vi "Drag and Drop - Initiating a Custom Drag.vi"() -> ()   [LabVIEW 2023]
doc: "Illustrates how to perform Drag and Drop operations from a custom source to a custom target."
panel:
  in  "Stop":bool
  in  "Plot to Drag":i32 min=0 max=4 step=1
  out "Target Waveform":dbl[](graph)
  out "Source Waveforms":dbl[][](graph)
  # "Overview: Demonstrates how to store the Mouse Down state and initiate custom drag operations when performing Drag and Drop actions with the Event Structure.\nInstructions:\n1. Run the VI.\n2. Specify a value for the Plot to Drag.\n3. Drag the plot area of the Source Waveforms graph to the Target Waveform graph. The specified Plot to Drag will appear in the Target Waveform.\n4. Click Stop to stop the VI."
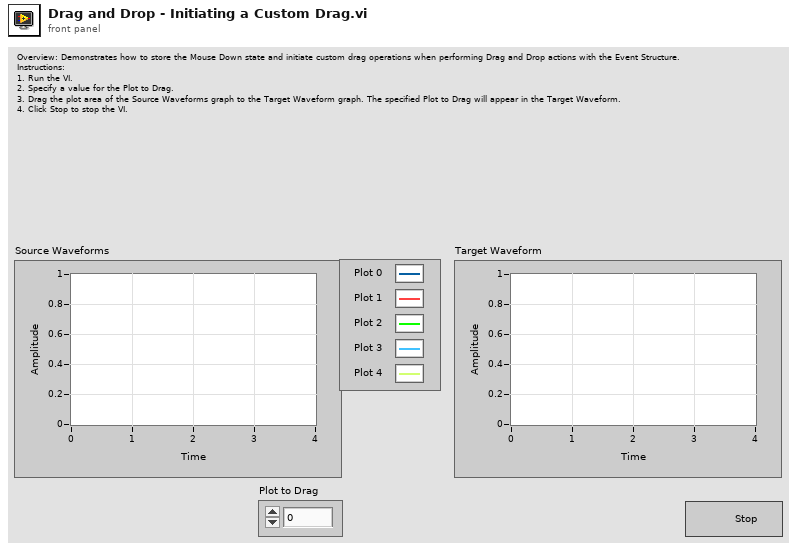
[diagram p1: front panel]
types:
  T1 = cluster{"data name":string, "drag data":variant}[]
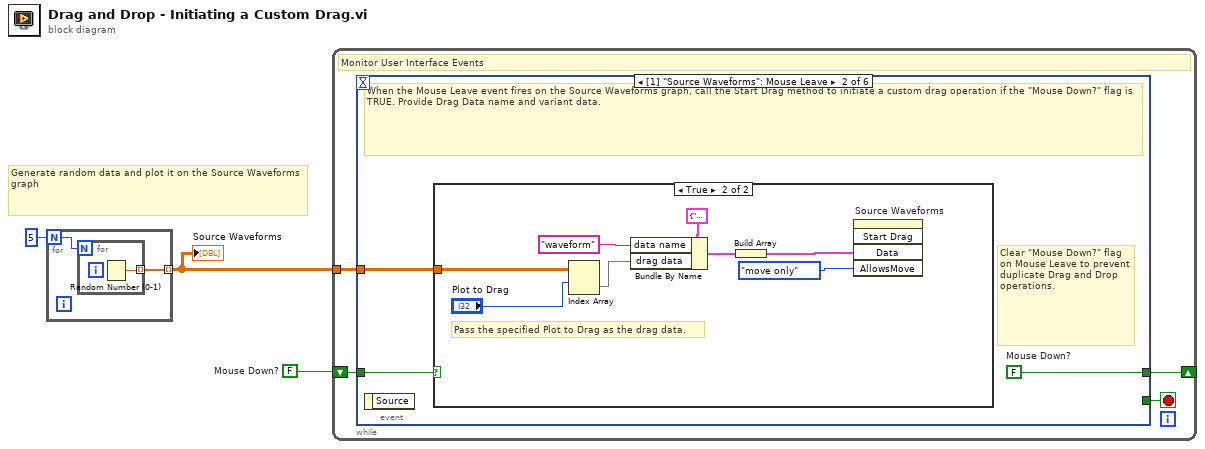
[diagram p0: block diagram]
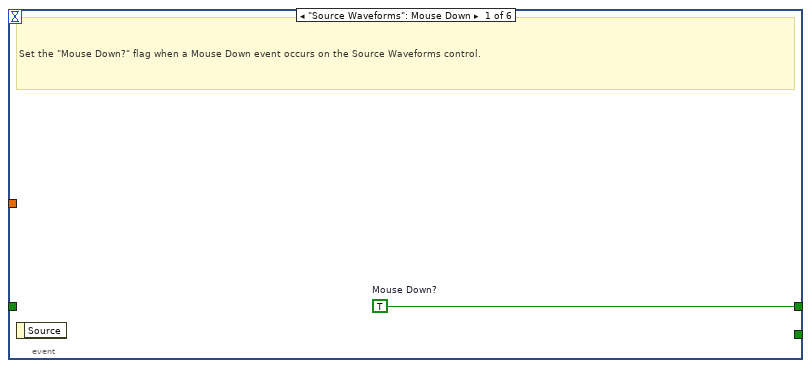
[diagram p2: hidden frame]
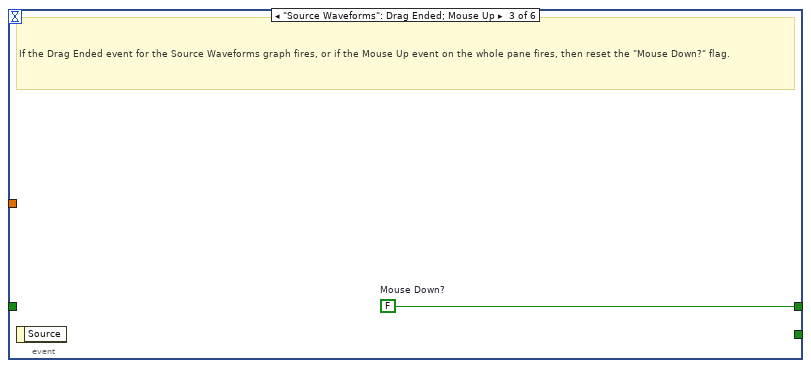
[diagram p4: hidden frame]
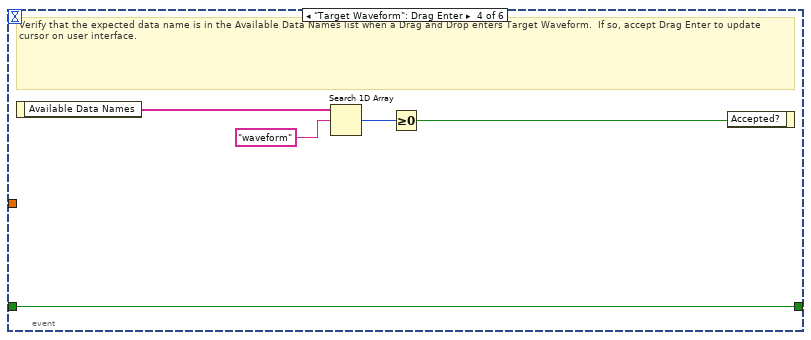
[diagram p5: hidden frame]
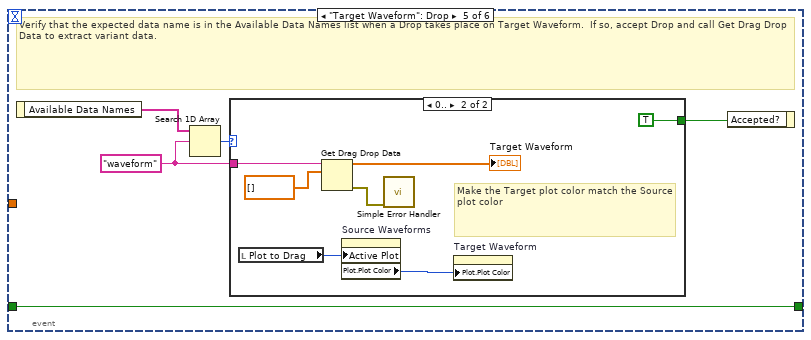
[diagram p6: hidden frame]
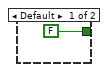
[diagram p7: hidden frame]
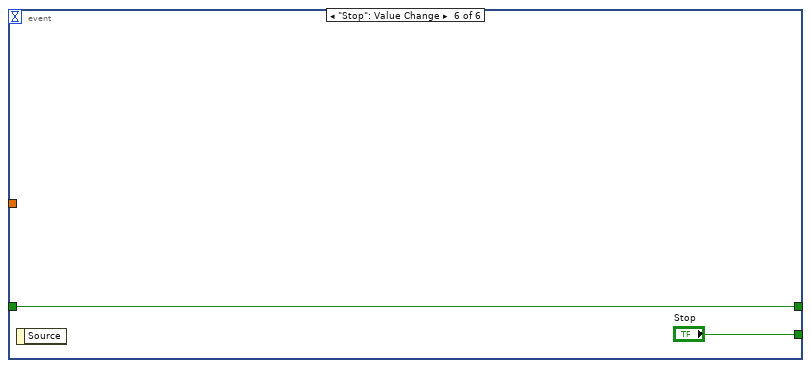
[diagram p8: hidden frame]
diagram:
  w2 = FALSE  # Mouse Down?
  # "Generate random data and plot it on the Source Waveforms graph"
  n1 = for {
    N: 5 -> [w4]
    tunnel: [w5] -> w3 mode=indexing
    n2 = for {
      N: w4 -> [_]
      tunnel: [w6] -> w5 mode=indexing
      n3 = Random Number (0-1)() -> (number: 0 to 1=w6:dbl)
    }
  }
  "Source Waveforms" <- w3
  n4 = while {
    tunnel: w3 -> [w10]
    shift-right: [w8] -> _
    shift-left: w2 -> [w9]
    stop <- w7 stop-if-true
    # "Monitor User Interface Events"
    n5 = event shown="[1] \"Source Waveforms\": Mouse Leave" {
      selector: _ -> [_ _ _ _ _ _]
      dyn-events: _ -> [_ _ _ _ _ _]
      timeout: _ -> [_ _ _ _ _ _]
      tunnel: w10 -> [_ w14 _ _ _ _]
      tunnel: w9 -> [_ w13 _ w25 w31 w42]
      tunnel: [w11 w12 w23 w25 w31 w42] -> w8
      tunnel: [_ _ _ _ _ "Stop"] -> w7
      event "Source Waveforms": Mouse Down {
        w11 = TRUE  # Mouse Down?
        # "Set the \"Mouse Down?\" flag when a Mouse Down event occurs on the Source Waveforms control."
        n6 = event-data() -> ()  [unwired: 1 in, 1 out]
      }
      event "Source Waveforms": Mouse Leave {
        w12 = FALSE  # Mouse Down?
        # "Clear \"Mouse Down?\" flag on Mouse Leave to prevent duplicate Drag and Drop operations."
        # "When the Mouse Leave event fires on the Source Waveforms graph, call the Start Drag method to initiate a custom drag operation if the \"Mouse Down?\" flag is TRUE. Provide Drag Data name and variant data."
        n7 = event-data() -> ()  [unwired: 1 in, 1 out]
        n8 = case shown="True" w13 {
          tunnel: w14 -> [_ w17]
          frame False {
          }
          frame True {
            # "Pass the specified Plot to Drag as the drag data."
            n9 = Index Array(array=w17, index (row)="Plot to Drag") -> (element=w16:dbl[])  [unwired: 1 in]
            n10 = Bundle By Name(cluster=cluster{"data name":string, "drag data":variant} {"data name"="", "drag data"=variant}, "data name"="waveform", "drag data"=w16) -> (w21:cluster{"data name":string, "drag data":variant})
            n11 = Build Array(w21) -> (w20:T1)
            n12 = invoke on="Source Waveforms" class="WFGraph (strict)" method="Start Drag"("Data"=w20, "AllowsMove"=enum32{"copy or move", "copy only", "move only"}."move only" ("Drag Mode")) -> ()  [unwired: 3 in, 5 out]
          }
        }
      }
      event "Source Waveforms": Drag Ended; Mouse Up {
        w23 = FALSE  # Mouse Down?
        # "If the Drag Ended event for the Source Waveforms graph fires, or if the Mouse Up event on the whole pane fires, then reset the \"Mouse Down?\" flag."
        n13 = event-data() -> ()  [unwired: 1 in, 1 out]
      }
      event "Target Waveform": Drag Enter {
        # "Verify that the expected data name is in the Available Data Names list when a Drag and Drop enters Target Waveform.  If so, accept Drag Enter to update cursor on user interface."
        n14 = event-data() -> ("Available Data Names"=w28:string[])  [unwired: 1 in]
        n15 = Search 1D Array(1D array=w28, element="waveform") -> (index of element=w24:i32)  [unwired: 1 in]
        n16 = Greater Or Equal To 0?(x=w24) -> (x >= 0?=w26:bool)
        n17 = event-data("Accepted?"=w26) -> ()  [unwired: 1 in, 1 out]
      }
      event "Target Waveform": Drop {
        w30 = "waveform" ("element")
        # "Verify that the expected data name is in the Available Data Names list when a Drop takes place on Target Waveform.  If so, accept Drop and call Get Drag Drop Data to extract variant data."
        n18 = event-data() -> ("Available Data Names"=w29:string[])  [unwired: 1 in]
        n19 = Search 1D Array(1D array=w29, element=w30) -> (index of element=w32:i32)  [unwired: 1 in]
        n20 = case shown="0.." w32 {
          tunnel: [FALSE TRUE] -> w33
          tunnel: w30 -> [_ w35]
          frame Default {
          }
          frame 0.. {
            # "Make the Target plot color match the Source plot color"
            n21 = local read "Plot to Drag"() -> (w37:i32)
            n22 = Get Drag Drop Data(8:dbl[] [], 9:w35) -> (0:w38:errorcluster, 3:→"Target Waveform":dbl[])  [unwired: 1 in]
            n23 = property on="Source Waveforms" class="WFGraph (strict)"("Active Plot"=w37) -> ("Plot.Plot Color"=w36:u32)  [unwired: 2 in, 2 out]
            n24 = call <vilib>:"Simple Error Handler.vi"("error in (no error)"=w38) -> ()  [unwired: 4 in, 5 out]
            n25 = property on="Target Waveform" class="WFGraph (strict)"("Plot.Plot Color"=w36) -> ()  [unwired: 2 in, 2 out]
          }
        }
        n26 = event-data("Accepted?"=w33) -> ()  [unwired: 1 in, 1 out]
      }
      event "Stop": Value Change {
        n27 = event-data() -> ()  [unwired: 1 in, 1 out]
      }
    }
  }
